vi "FTW-JSON-Object-Keys.vi"(0 "JSON Object":refnum<class "FTW-JSON.lvclass">, 11 "error in":errorcluster) -> (4 "JSON Object out":refnum<class "FTW-JSON.lvclass">, 6 "Keys":string[](array[string]), 8 "Elements":i64[](array[numeric]) format="%016x", 15 "error out":errorcluster)   [LabVIEW 2013, in "FTW-JSON.lvclass"]
uses:
  FTW-JSON.lvclass
  FTW-JSON.lvclass/FTW-JSON.ctl
panel:
  # "Inputs"
  # "Outputs"
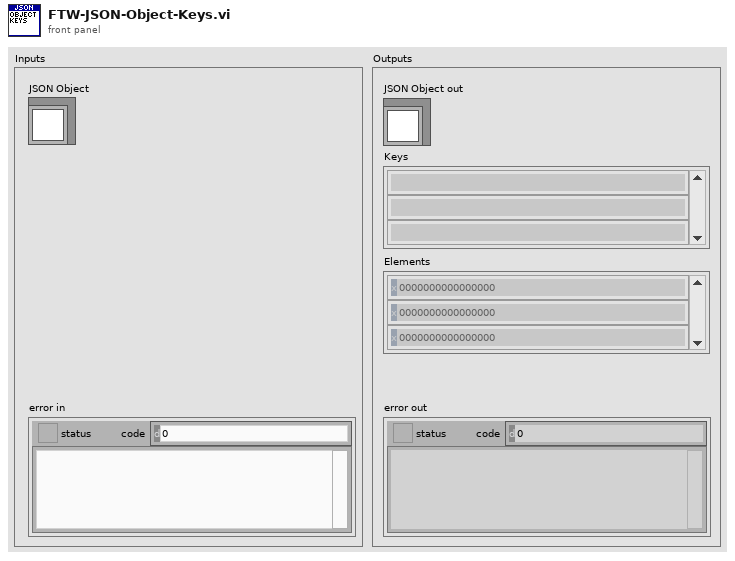
[diagram p1: front panel]
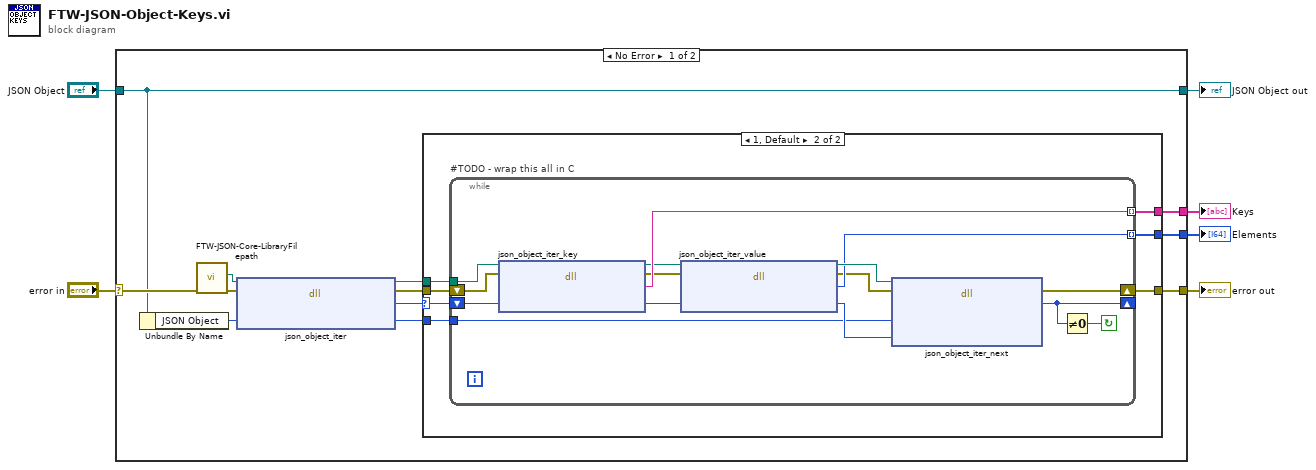
[diagram p0: block diagram]
diagram:
  n1 = case shown="No Error" "error in" {
    selector: "error in" -> [w14 w43]
    tunnel: [w18 w43] -> w6
    tunnel: [w9 w42] -> w4
    tunnel: "JSON Object" -> [w9 w42]
    tunnel: [w17 _] -> w2
    tunnel: [w16 _] -> w1
    frame No Error {
      n2 = Unbundle By Name(w9) -> ("JSON Object"=w11:i64)
      n3 = call "FTW-JSON-Core-LibraryFilepath.vi"("error in"=w14) -> ("error out"=w13:errorcluster, "JSON Library Filepath"=w12:path)  [unwired: 9 in]
      n4 = dll-call lib="?" fn="json_object_iter"(path in=w12, error in=w13, "JSON Object Pointer"=w11) -> (path out=w8:path, error out=w15:errorcluster, "JSON Object Iterator Pointer"=w7:i64, "JSON Object Pointer"=w10:i64)  [unwired: 1 in]
      n5 = case shown="1, Default" w7 {
        selector: w7 -> [_ w20]
        tunnel: [w19 w26] -> w18
        tunnel: [_ w25] -> w17
        tunnel: [_ w24] -> w16
        tunnel: w15 -> [w19 w23]
        tunnel: w10 -> [_ w22]
        tunnel: w8 -> [_ w21]
        frame 0 {
        }
        frame 1, Default {
          n6 = while "#TODO - wrap this all in C" {
            tunnel: [w40] -> w24 mode=indexing
            tunnel: [w29] -> w25 mode=indexing
            shift-right: [w41] -> w26
            shift-left: w23 -> [w32]
            tunnel: w22 -> [w34]
            tunnel: w21 -> [w33]
            shift-right: [w30] -> _
            shift-left: w20 -> [w31]
            stop <- w27 continue-if-true
            n7 = dll-call lib="?" fn="json_object_iter_key"(path in=w33, error in=w32, "JSON Iterator Pointer"=w31) -> (path out=w38:path, error out=w37:errorcluster, "Current Key"=w40:string, "JSON Iterator Pointer"=w36:i64)  [unwired: 1 in]
            n8 = dll-call lib="?" fn="json_object_iter_value"(path in=w38, error in=w37, "JSON Iterator Pointer"=w36) -> (path out=w35:path, error out=w28:errorcluster, "JSON Object Pointer"=w29:i64, "JSON Iterator Pointer"=w39:i64)  [unwired: 1 in]
            n9 = dll-call lib="?" fn="json_object_iter_next"(path in=w35, error in=w28, "JSON Object Pointer"=w34, "JSON Iterator Pointer"=w39) -> (error out=w41:errorcluster, "Next JSON Iterator Pointer"=w30:i64)  [unwired: 3 in, 1 out]
            n10 = Not Equal To 0?(x=w30) -> (x != 0?=w27:bool)
          }
        }
      }
    }
    frame Error {
    }
  }
  "error out" <- w6
  "JSON Object out" <- w4
  "Elements" <- w2
  "Keys" <- w1
